vi "二极管伏安特性曲线.vi"() -> ()   [LabVIEW 2020]
uses:
  <vilib>/Analysis/baseanly.llb/Mean (DBL).vi
  <vilib>/Analysis/NI_AALBase.lvlib
panel:
  out "数据":dbl[][](array[numeric])
  in  "电压上限(V)":dbl
  in  "电压递增步长(V)":dbl
  in  "采集时间间隔":dbl[unit]
  in  "标准电阻值(欧姆)":dbl
  in  "开关":bool
  out "电阻的伏安特性曲线":cluster{"Y":dbl[], "Y":dbl[]}[](graph)=[{"Y"=[-7.891009970234075e-05, 0.22745491335365312, 0.45497526249279086, 0.6824788494493705, 0.9097322315434345, 1.1373568233619646, 1.365040270759496, 1.5925951653865802, 1.8199919139109821, 2.047414637757974, 2.274922519009644, 2.50271282775536, 2.730029353204874, 2.9574869264537877, 3.184924442494402, 3.412588487178624, 3.6401502769725886, 3.8676262471396328, 4.095069006955003, 4.322537732914449, 4.550144211953193], "Y"=[3.210967070956557e-05, 0.00025628009886622424, 0.000482554769784973, 0.0007067251455556644, 0.0009321120253810415, 0.001155657644255959, 0.001380945833999103, 0.001604327004870657, 0.001828727404327643, 0.002053653844402069, 0.002277988433133287, 0.0025028161831974916, 0.0027273479945272854, 0.0029521099337520397, 0.0031761813844617837, 0.0034011734252725264, 0.0036252119444909296, 0.003850236811877774, 0.004074143762180228, 0.0042988397856283025, 0.00452360154105194]}]
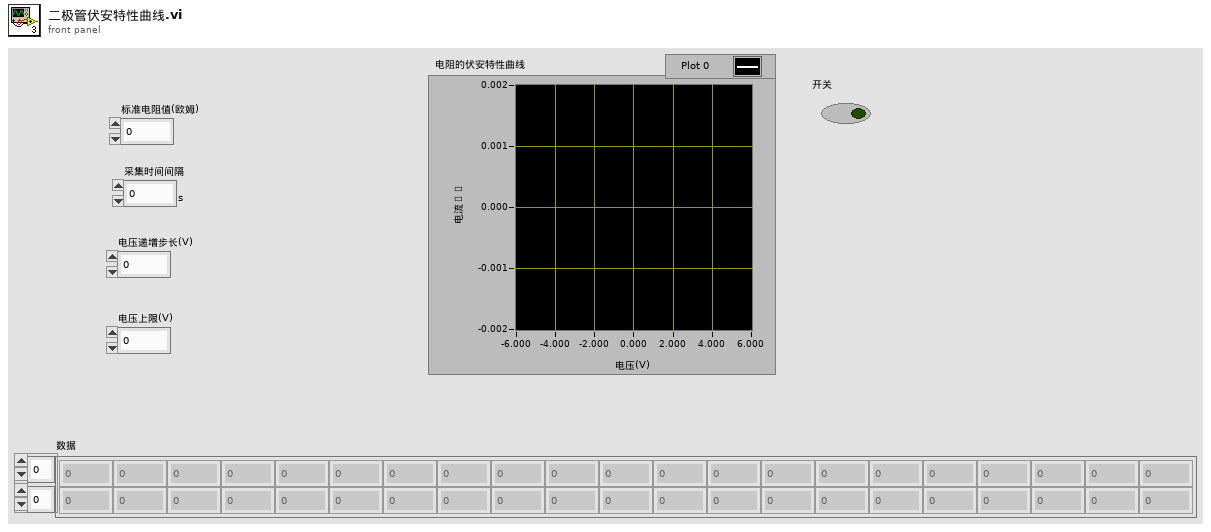
[diagram p1: front panel]
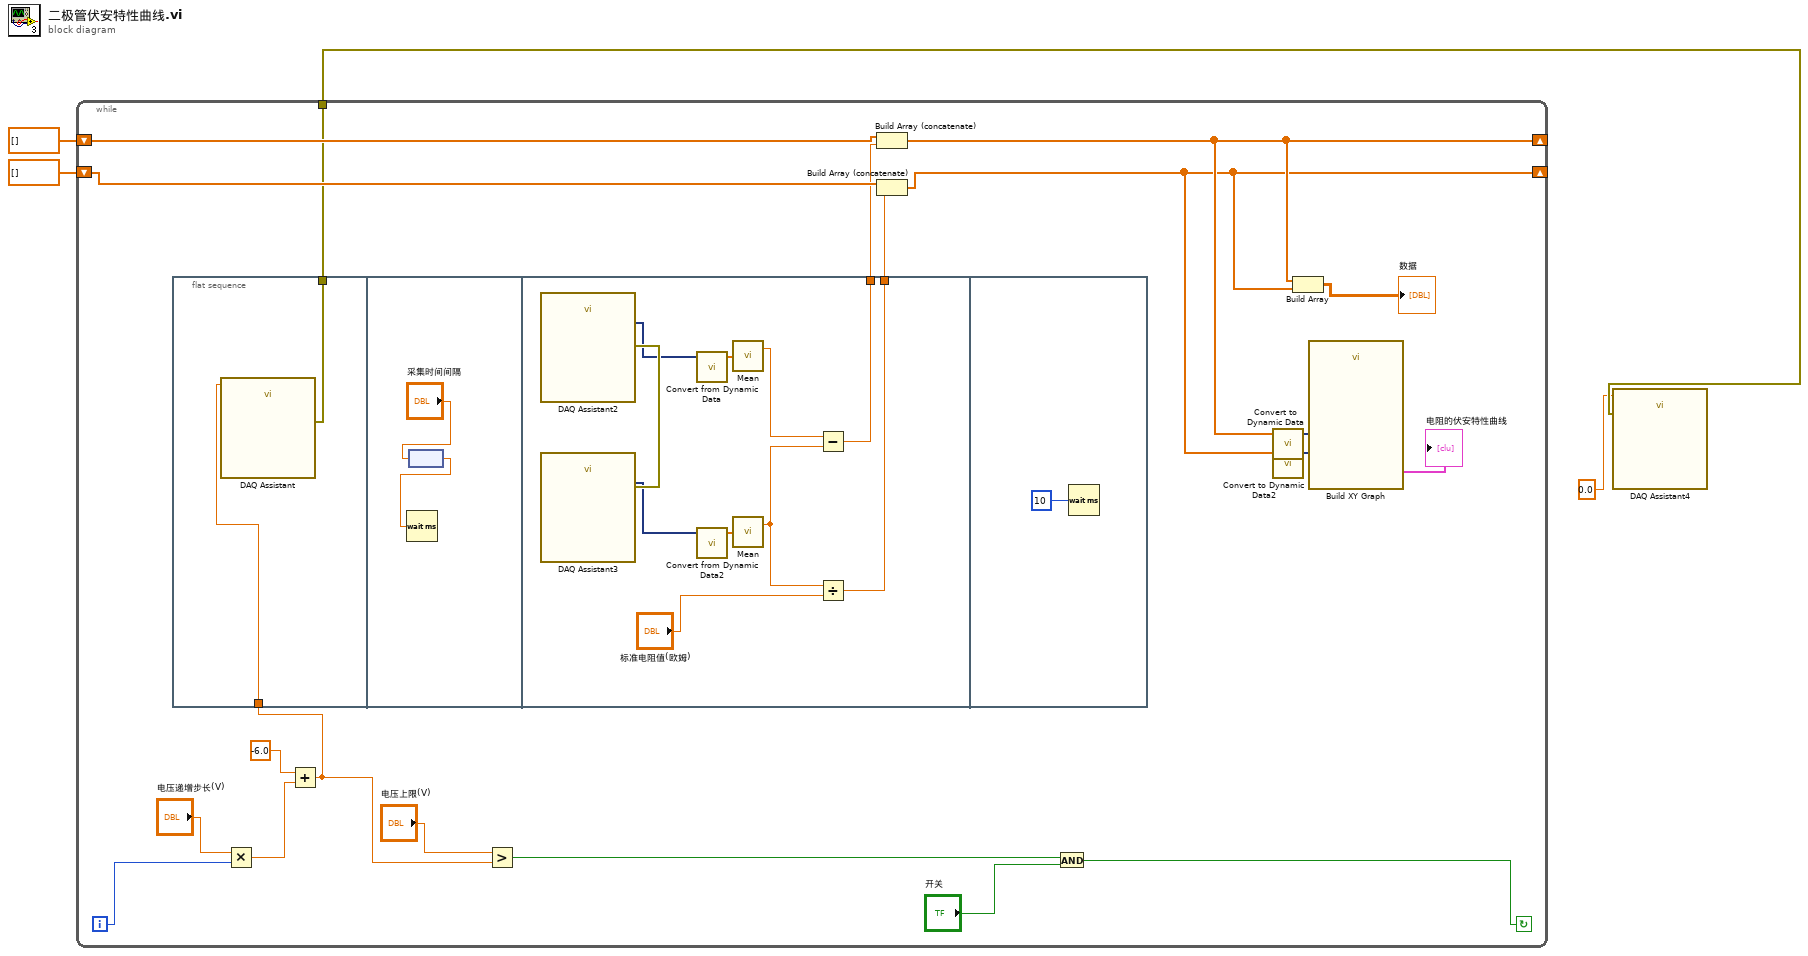
[diagram p0: block diagram]
diagram:
  n1 = while {
    shift-right: [w12] -> _
    shift-left: dbl[] [] -> [w17]
    shift-right: [w10] -> _
    shift-left: dbl[] [] -> [w16]
    tunnel: [w8] -> w2
    i -> [w22]
    stop <- w18 continue-if-true
    n2 = flat-sequence {
      tunnel: w5 -> [w26]
      tunnel: [w25] -> w8
      tunnel: [w30] -> w15
      tunnel: [w29] -> w14
      frame #0 {
        n3 = call "DAQ Assistant"("data"=w26) -> ("error out"=w25:errorcluster)  [unwired: 17 in, 1 out]
      }
      frame #1 {
        n4 = node("采集时间间隔") -> (w27:dbl)
        n5 = Wait (ms)(milliseconds to wait=w27) -> ()  [unwired: 1 out]
      }
      frame #2 {
        n6 = call "DAQ Assistant2"() -> ("data"=w37:dynamicdata, "error out"=w38:errorcluster)  [unwired: 17 in, 1 out]
        n7 = call "DAQ Assistant3"("error in"=w38) -> ("data"=w35:dynamicdata)  [unwired: 16 in, 2 out]
        n8 = call "Convert from Dynamic Data"("Dynamic Data Type"=w37) -> ("Array"=w36:dbl[])  [unwired: 3 in]
        n9 = call "Convert from Dynamic Data2"("Dynamic Data Type"=w35) -> ("Array"=w34:dbl[])  [unwired: 3 in]
        n10 = call-poly <vilib>:"Mean.vi"("X"=w36) -> ("mean"=w32:dbl)  [unwired: 1 out]
        n11 = call-poly <vilib>:"Mean.vi"("X"=w34) -> ("mean"=w31:dbl)  [unwired: 1 out]
        n12 = Subtract(x=w32, y=w31) -> (x-y=w30:dbl)
        n13 = Divide(x=w31, y="标准电阻值(欧姆)") -> (x/y=w29:dbl)
      }
      frame #3 {
        n14 = Wait (ms)(milliseconds to wait=u32 10) -> ()  [unwired: 1 out]
      }
    }
    n15 = Multiply(x="电压递增步长(V)", y=w22) -> (x*y=w7:dbl)
    n16 = Add(x=-6.0, y=w7) -> (x+y=w5:dbl)
    n17 = Greater?(x="电压上限(V)", y=w5) -> (0:w19:bool)
    n18 = Build Array (concatenate) "Build Array"(w17, w15) -> (w12:dbl[])
    n19 = Build Array (concatenate) "Build Array"(w16, w14) -> (w10:dbl[])
    n20 = And(x=w19, y="开关") -> (x .and. y?=w18:bool)
    n21 = call "Convert to Dynamic Data"("Array"=w12) -> ("Dynamic Data Type"=w11:dynamicdata)  [unwired: 3 in]
    n22 = call "Convert to Dynamic Data2"("Array"=w10) -> ("Dynamic Data Type"=w9:dynamicdata)  [unwired: 3 in]
    n23 = Build Array "Build Array"(w12, w10) -> (→"数据":dbl[][])
    n24 = call "Build XY Graph"("Y Input"=w9, "X Input"=w11) -> ("XY Graph"=→"电阻的伏安特性曲线":cluster{"X":dbl[], "Y":dbl[]}[])  [unwired: 8 in, 1 out]
  }
  n25 = call "DAQ Assistant4"("data"=0.0, "error in"=w2) -> ()  [unwired: 16 in, 2 out]
